vi "Stop Core.vi"(10 "final error code":i32, 11 "Nested in":refnum<class "Chart Actor.lvclass">) -> (3 "Nested out":refnum<class "Chart Actor.lvclass">)   [LabVIEW 2018, in "Chart Actor.lvlib" / "Chart Actor.lvclass"]
uses:
  Chart Actor.lvclass
  <vilib>/MGI/Panel Manager/Panel Actor/Panel Actor/Panel Actor.lvclass
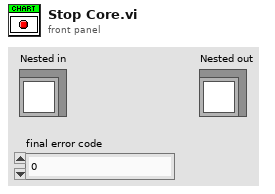
[diagram p1: front panel]
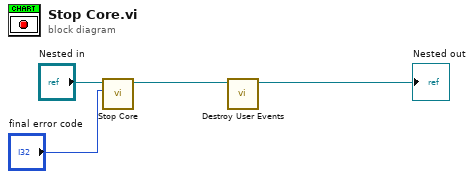
[diagram p0: block diagram]
diagram:
  n1 = call-parent "Stop Core.vi"("final error code"="final error code", "Monitored Actor in"="Nested in") -> ("Monitored Actor out"=w2:refnum<class "Chart Actor.lvclass">)  [unwired: 9 in]
  n2 = call "Destroy User Events.vi"("UI Template in"=w2) -> ("UI Template out"=→"Nested out":refnum<class "Chart Actor.lvclass">)  [unwired: 10 in]
